vi "Setrelay_action.vi"(8 "error in (no error)":errorcluster, 10 "Set_Val":T1, 11 "OneOfTemplate in":refnum<class "niswitch_grpc_RelayControlRequest_relay_action_enum.lvclass">) -> (0 "error out":errorcluster, 3 "OneOfTemplate out":refnum<class "niswitch_grpc_RelayControlRequest_relay_action_enum.lvclass">)   [LabVIEW 2021, in "NI Switch_client.lvlib" / "niswitch_grpc_RelayControlRequest_relay_action_enum.lvclass"]
uses:
  niswitch_grpc_RelayControlRequest_relay_action_enum.lvclass
  niswitch_grpc_RelayControlRequest_relay_action_enum.lvclass/niswitch_grpc_RelayControlRequest_relay_action_enum.ctl
  niswitch_grpc_RelayAction.ctl
  NI Switch_client.lvlib
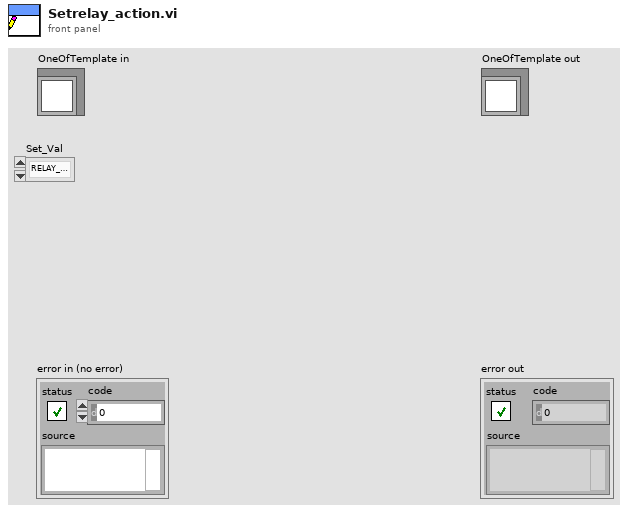
[diagram p1: front panel]
types:
  T1 = typedef "NI Switch_client.lvlib/niswitch_grpc_RelayAction.ctl" = enum32{"RELAY_ACTION_UNSPECIFIED", "RELAY_ACTION_NISWITCH_VAL_OPEN_RELAY", "RELAY_ACTION_NISWITCH_VAL_CLOSE_RELAY"}
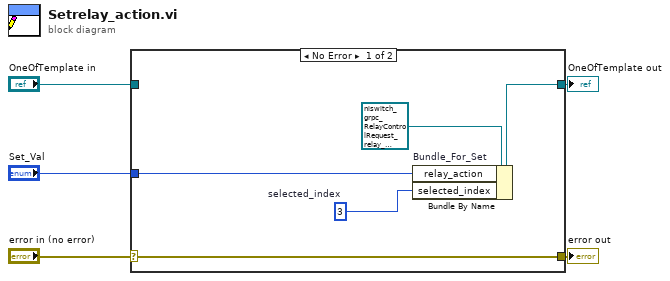
[diagram p0: block diagram]
diagram:
  n1 = case shown="No Error" "error in (no error)" {
    selector: "error in (no error)" -> [w10 w11]
    tunnel: [w10 w11] -> w4
    tunnel: [w9 w12] -> w2
    tunnel: "OneOfTemplate in" -> [_ w12]
    tunnel: "Set_Val" -> [w8 _]
    frame No Error {
      w7 = 3  # selected_index
      n2 = Bundle By Name "Bundle_For_Set"(cluster=refnum<class "niswitch_grpc_RelayControlRequest_relay_action_enum.lvclass"> refnum ("OneOfTemplate in"), "relay_action"=w8, "selected_index"=w7) -> (w9:refnum<class "niswitch_grpc_RelayControlRequest_relay_action_enum.lvclass">)
    }
    frame Error {
    }
  }
  "error out" <- w4
  "OneOfTemplate out" <- w2
